vi "APS get int factor.vi"(7 "Enable":i32, 8 "error in (no error)":errorcluster caption="错误输入（无错误）", 9 "Factor_No":i32, 10 "Item_No":i32, 11 "Board_ID":i32) -> (0 "error out":errorcluster caption="错误输出", 3 "function return":i32, 5 "Enable out":i32)   [LabVIEW 2011, in "APS168.lvlib"]
doc: "I32 FNTYPE APS_get_int_factor( I32 Board_ID, I32 Item_No, I32 Factor_No, I32 *Enable );"
uses:
  APS168.lvlib
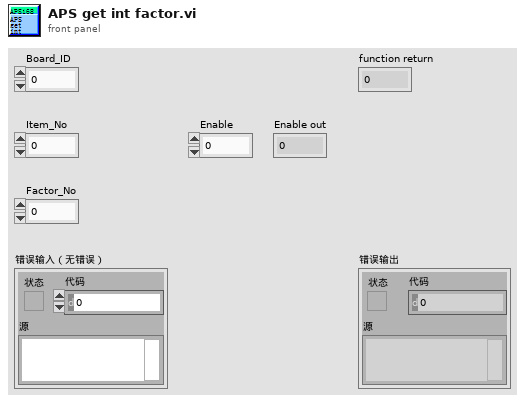
[diagram p1: front panel]
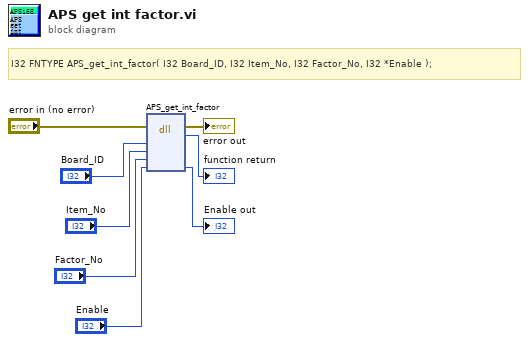
[diagram p0: block diagram]
diagram:
  # "I32 FNTYPE APS_get_int_factor( I32 Board_ID, I32 Item_No, I32 Factor_No, I32 *Enable );"
  n1 = dll-call lib="PTH1Labs E软件ADLINK 204CAPS_1_7_1_LIB line 连续运动204APS168.*" fn="APS_get_int_factor"(error in="error in (no error)", "Board_ID"="Board_ID", "Item_No"="Item_No", "Factor_No"="Factor_No", "Enable"="Enable") -> (error out=→"error out":errorcluster, →"function return":i32, "Enable"=→"Enable out":i32)  [unwired: 5 in, 1 out]
